vi "Exercise1.0-Basic Data Type.vi"() -> ()   [LabVIEW 2013]
panel:
  out "Tank":dbl(slide) scale=0.0..10.0
  out "Meter":dbl(knob) scale=0.0..10.0
  in  "Boolean":bool
  in  "Knob":dbl(knob) scale=0.0..10.0
  in  "Slide":dbl(slide) scale=0.0..10.0
  out "String Output":string
  in  "String Input":string
  in  "Boolean Input":bool
  out "Boolean Output":bool
  out "Numeric Output":dbl
  in  "Numeric Input":dbl
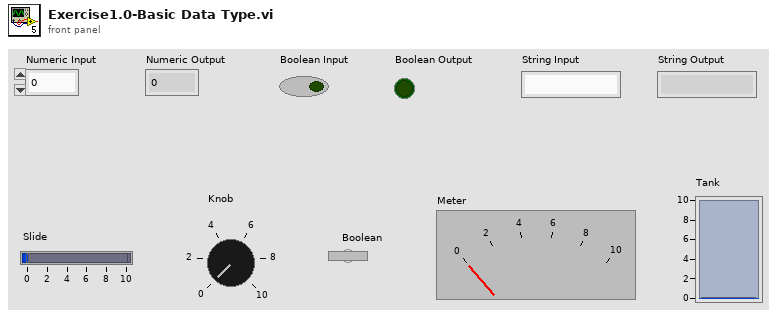
[diagram p1: front panel]
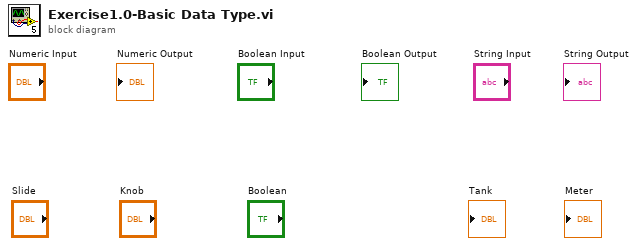
[diagram p0: block diagram]
diagram:
